vi "Write Mods.vi"(8 "error in (no error)":errorcluster, 10 "Mods":cluster{"Double Click":bool, "Menu Key":bool}, 11 "Handle Click on Graph Msg in":refnum<class "Handle Click on Graph Msg.lvclass">) -> (0 "error out":errorcluster, 3 "Handle Click on Graph Msg out":refnum<class "Handle Click on Graph Msg.lvclass">)   [LabVIEW 2020, in "GarphView.lvlib" / "Handle Click on Graph Msg.lvclass"]
uses:
  Handle Click on Graph Msg.lvclass
  Handle Click on Graph Msg.lvclass/Handle Click on Graph Msg.ctl
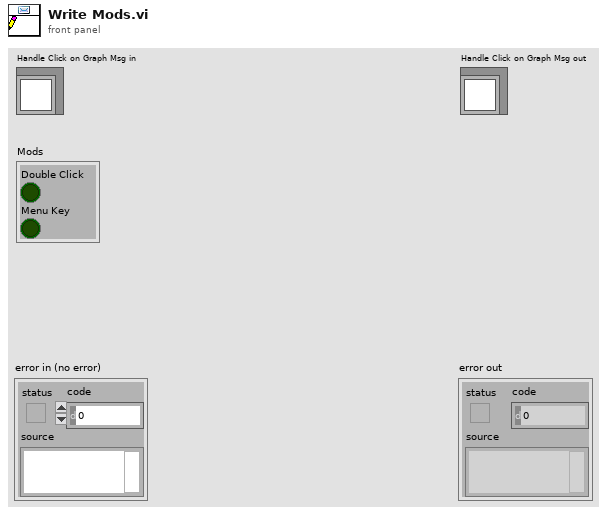
[diagram p1: front panel]
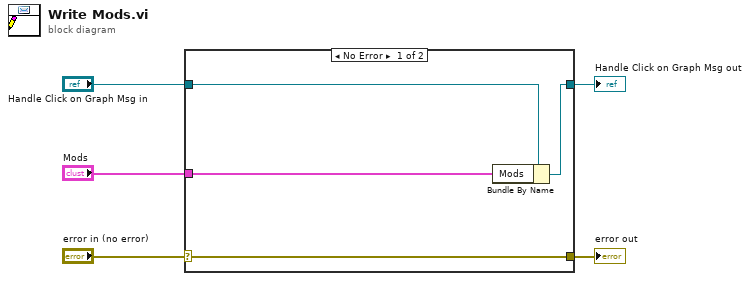
[diagram p0: block diagram]
diagram:
  n1 = case shown="No Error" "error in (no error)" {
    selector: "error in (no error)" -> [w9 w10]
    tunnel: [w9 w10] -> w4
    tunnel: [w7 w11] -> w2
    tunnel: "Handle Click on Graph Msg in" -> [w8 w11]
    tunnel: "Mods" -> [w6 _]
    frame No Error {
      n2 = Bundle By Name(cluster=w8, "Mods"=w6) -> (w7:refnum<class "Handle Click on Graph Msg.lvclass">)
    }
    frame Error {
    }
  }
  "error out" <- w4
  "Handle Click on Graph Msg out" <- w2
